vi "Reference Init.vi"(3 "Container State":T3, 4 "Previous State":variant=variant(cluster{"State":enum16{"Initialized", "First Run"}} {"State"=enum."Initialized"}), 5 "Previous Version":T2={"Major"=1, "Minor"=0, "Fix"=0, "Build"=0}) -> (2 "Current State":T1)   [LabVIEW 2016, in "VI Reference.xctl"]
uses:
  VI Reference.xctl
  Reference State.ctl
  VI Reference Control/VI Reference Control.lvclass
  <vilib>/_xctls/Container State.ctl
  <vilib>/_xctls/Version.ctl
  <vilib>/_xctls/XControlSupport.lvlib
panel:
  in  "Current State":T1 caption="Default Indicator State"
  in  "Current State":T1 caption="Default Control State"
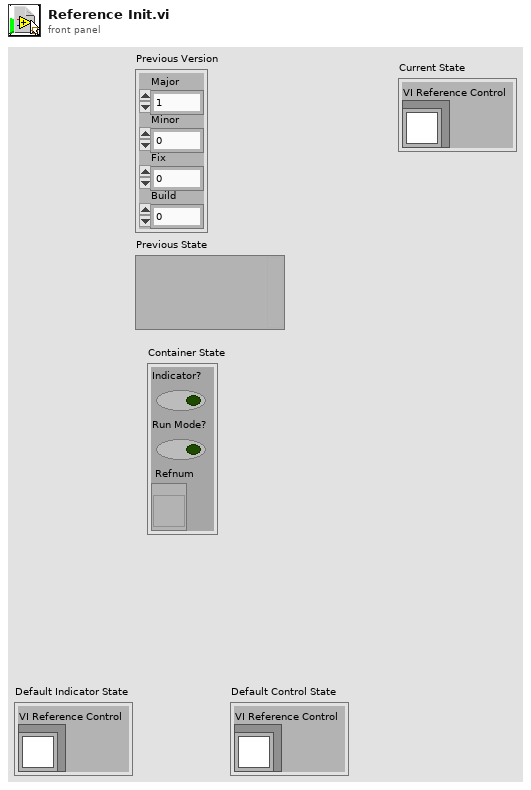
[diagram p1: front panel]
types:
  T1 = typedef "VI Reference.xctl/Reference State.ctl" = cluster{"VI Reference Control":refnum<class "VI Reference Control.lvclass">}
  T2 = typedef "XControlSupport.lvlib/Version.ctl" = cluster{"Major":u16, "Minor":u16, "Fix":u16, "Build":u16}
  T3 = typedef "XControlSupport.lvlib/Container State.ctl" = cluster{"Indicator?":bool, "Run Mode?":bool, " Refnum":refnum<vi>}
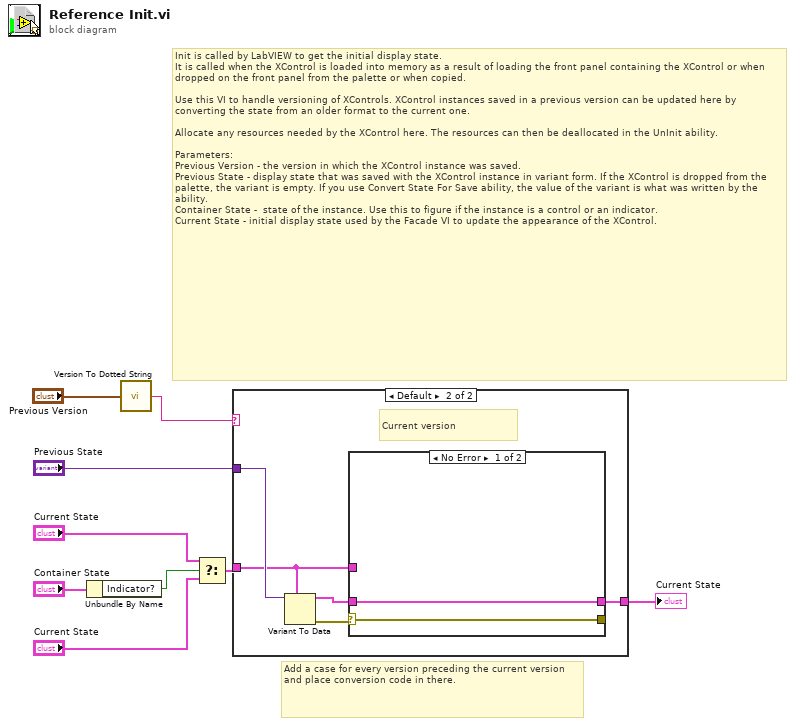
[diagram p0: block diagram]
diagram:
  # "Add a case for every version preceding the current version and place conversion code in there."
  # "Init is called by LabVIEW to get the initial display state.\nIt is called when the XControl is loaded into memory as a result of loading the front panel containing the XControl or when dropped on the front panel from the palette or when copied.\n\nUse this VI to handle versioning of XControls. XControl instances saved in a previous version can be updated here by converting the state from an older format to the current one.\n\nAllocate any resources needed by the XControl here. The resources can then be deallocated in the UnInit ability.\n\nParameters:\nPrevious Version - the version in which the XControl instance was saved.\nPrevious State - display state that was saved with the XControl instance in variant form. If the XControl is dropped from the palette, the variant is empty. If you use Convert State For Save ability, the value of the variant is what was written by the ability. \nContainer State -  state of the instance. Use this to figure if the instance is a control or an indicator.\nCurrent State - initial display state used by the Facade VI to update the appearance of the XControl."
  n1 = Unbundle By Name("Container State") -> ("Indicator?"=w5:bool)
  n2 = call <vilib>:"Version To Dotted String.vi"("Version"="Previous Version") -> ("String Version"=w2:string)
  n3 = Select(t="Current State", s=w5, f="Current State") -> (s? t:f=w4:T1)
  n4 = case shown="Default" w2 {
    tunnel: "Previous State" -> [_ w15]
    tunnel: [w10 w11] -> w1
    tunnel: w4 -> [w10 w12]
    frame "0.0.0.0" {
      # "Just created, use default state"
    }
    frame Default {
      # "Current version"
      n5 = Variant To Data(type=w12, Variant=w15) -> (data=w13:T1, error out=w14:errorcluster)  [unwired: 1 in]
      n6 = case shown="No Error" w14 {
        selector: w14 -> [w17 w18]
        tunnel: w13 -> [w16 _]
        tunnel: [w16 w19] -> w11
        tunnel: w12 -> [_ w19]
        tunnel: [w17 w18] -> _
        frame No Error {
        }
        frame Error {
          # "Error converting previously \nsaved state. Use default instead."
        }
      }
    }
  }
  "Current State" <- w1
